vi "Execute application.vi"(0 "Browser":string(combo)="Edge", 5 "Mode":string(combo), 7 "Website URL":string="https://www.solitontech.com/", 11 "Error in":errorcluster) -> (15 "Error out":errorcluster)   [LabVIEW 2020, in "LV Connectivity.lvlib"]
doc: "This VI is used to open any website on browser selected user can select the browser and mode and can provide the URL they need to open."
uses:
  LV Connectivity.lvlib
panel:
  # "OPEN APPLICATION"
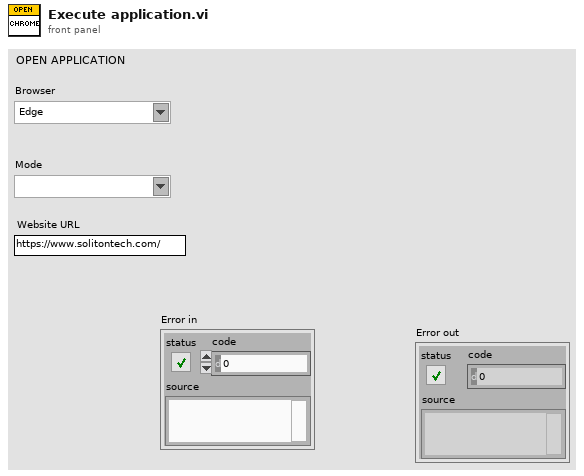
[diagram p1: front panel]
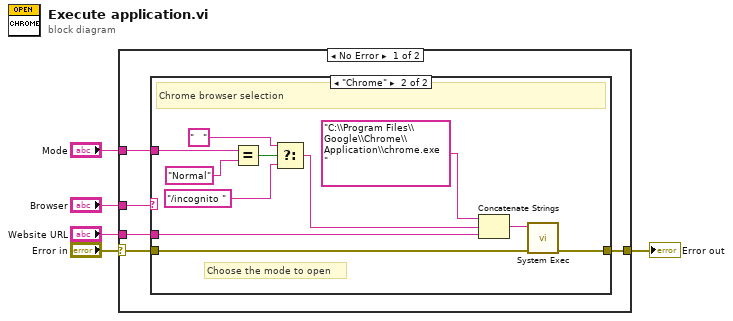
[diagram p0: block diagram]
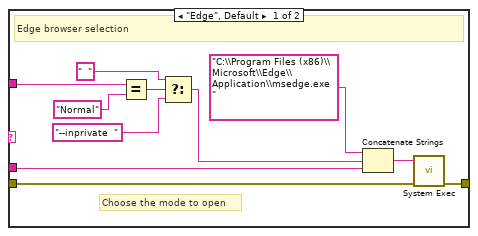
[diagram p2: hidden frame]
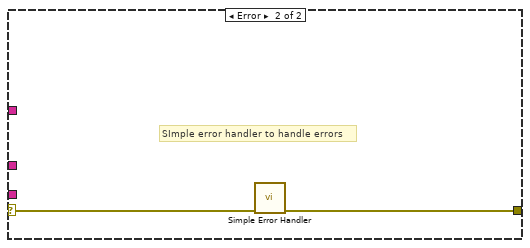
[diagram p3: hidden frame]
diagram:
  n1 = case shown="No Error" "Error in" {
    selector: "Error in" -> [w9 w34]
    tunnel: [w10 w33] -> w5
    tunnel: "Browser" -> [w8 _]
    tunnel: "Mode" -> [w7 _]
    tunnel: "Website URL" -> [w6 _]
    frame No Error {
      n2 = case shown="\"Chrome\"" w8 {
        tunnel: [w20 w32] -> w10
        tunnel: w9 -> [w21 w31]
        tunnel: w7 -> [w11 w30]
        tunnel: w6 -> [w13 w23]
        frame "Edge", Default {
          # "Choose the mode to open"
          # "Edge browser selection"
          n3 = Equal?(x=w11, y="Normal") -> (x = y?=w18:bool)
          n4 = Select(t="  ", s=w18, f="--inprivate  ") -> (s? t:f=w14:string)
          n5 = Concatenate Strings("C:\\Program Files (x86)\\Microsoft\\Edge\\Application\\msedge.exe  ", w14, w13) -> (w12:string)
          n6 = call <vilib>:"System Exec.vi"("error in (no error)"=w21, "command line"=w12) -> ("error out"=w20:errorcluster)  [unwired: 6 in, 3 out]
        }
        frame "Chrome" {
          # "Choose the mode to open"
          # "Chrome browser selection"
          n7 = Equal?(x=w30, y="Normal") -> (x = y?=w28:bool)
          n8 = Select(t="   ", s=w28, f="/incognito ") -> (s? t:f=w24:string)
          n9 = Concatenate Strings("C:\\Program Files\\Google\\Chrome\\Application\\chrome.exe  ", w24, w23) -> (w22:string)
          n10 = call <vilib>:"System Exec.vi"("error in (no error)"=w31, "command line"=w22) -> ("error out"=w32:errorcluster)  [unwired: 6 in, 3 out]
        }
      }
    }
    frame Error {
      # "SImple error handler to handle errors"
      n11 = call <vilib>:"Simple Error Handler.vi"("error in (no error)"=w34) -> ("error out"=w33:errorcluster)  [unwired: 4 in, 4 out]
    }
  }
  "Error out" <- w5
